vi "Append Report Text (num).vi"(0 "report in":refnum<class "NI_Excel.lvclass">, 1 "MS Office parameters":T1, 2 "format string (%.3f)":string="%.3f", 7 "text":dbl format="%.2f", 9 "append on new line? (F)":bool, 11 "error in (no error)":errorcluster) -> (4 "report out":refnum<class "NI_Excel.lvclass">, 8 "start out (Word)":i32, 10 "end out (Word)":i32, 15 "error out":errorcluster)   [LabVIEW 2023, in "NI_Excel.lvclass"]
doc: "Appends text to the selected report."
uses:
  NI_Excel.lvclass
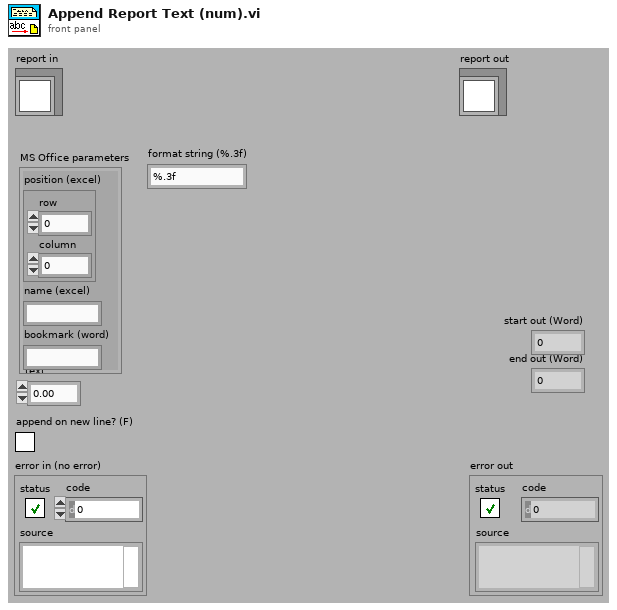
[diagram p1: front panel]
types:
  T1 = cluster{"position (excel)":cluster{"row":i32, "column":i32}, "name (excel)":string, "bookmark (word)":string}
  T2 = typedef "NI_ReportGenerationCore.lvlib/Report Data Members.ctl" = cluster{"font":T3, "from template?":bool}
  T3 = typedef "NI_ReportGenerationCore.lvlib/font.ctl" = cluster{"font name":string, "font size":dbl, "bold":u16, "italic":u16, "underline":u16, "strike through":u16, "font color":u32}
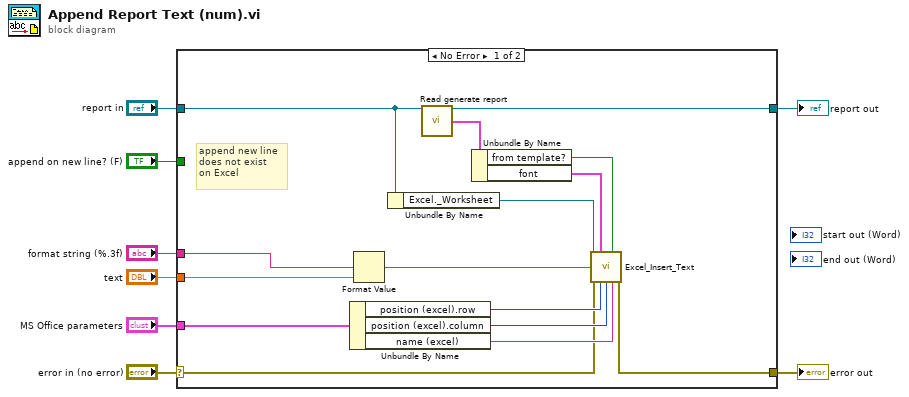
[diagram p0: block diagram]
diagram:
  n1 = case shown="No Error" "error in (no error)" {
    selector: "error in (no error)" -> [w15 w25]
    tunnel: [w14 w25] -> w7
    tunnel: [w12 w24] -> w5
    tunnel: "report in" -> [w13 w24]
    tunnel: "append on new line? (F)" -> [_ _]
    tunnel: "MS Office parameters" -> [w18 _]
    tunnel: "text" -> [w17 _]
    tunnel: "format string (%.3f)" -> [w16 _]
    frame No Error {
      # "append new line\ndoes not exist\non Excel"
      n2 = Unbundle By Name(w18) -> ("position (excel).row"=w22:i32, "position (excel).column"=w23:i32, "name (excel)"=w19:string)
      n3 = Format Value(format string=w16, value (0)=w17) -> (output string=w21:string)  [unwired: 1 out]
      n4 = Unbundle By Name(w13) -> ("Excel._Worksheet"=w20:refnum<k7>)
      n5 = call-dynamic "Read generate report.vi"("report in"=w13) -> ("report out"=w12:refnum<class "NI_Excel.lvclass">, "generate report"=w11:T2)  [unwired: 12 in, 1 out]
      n6 = Unbundle By Name(w11) -> ("from template?"=w10:bool, "font"=w9:T3)
      n7 = call <vilib>:"Excel_Insert_Text.vi"("worksheet"=w20, "font"=w9, "from template?"=w10, "value"=w21, "error in (no error)"=w15, "row"=w22, "column"=w23, "name"=w19) -> ("error out"=w14:errorcluster)  [unwired: 7 out]
    }
    frame Error {
    }
  }
  "error out" <- w7
  "report out" <- w5
